vi "Write Device Details.vi"(8 "error in":errorcluster, 10 "Device Details":T1={"Device Port Number"=2001, "Device IP"="192.168.1.1.100", "Timeout"=5000, "Port Number"=1234, "Connection ID"=refnum}, 11 "UDP in":refnum<class "UDP.lvclass">) -> (0 "error out":errorcluster, 3 "UDP out":refnum<class "UDP.lvclass">)   [LabVIEW 2020, in "Plugin Instrument Driver.lvlib" / "UDP.lvclass"]
doc: "Write Device Details"
uses:
  UDP.lvclass
  Typedefs/Device Details.ctl
  UDP.lvclass/UDP.ctl
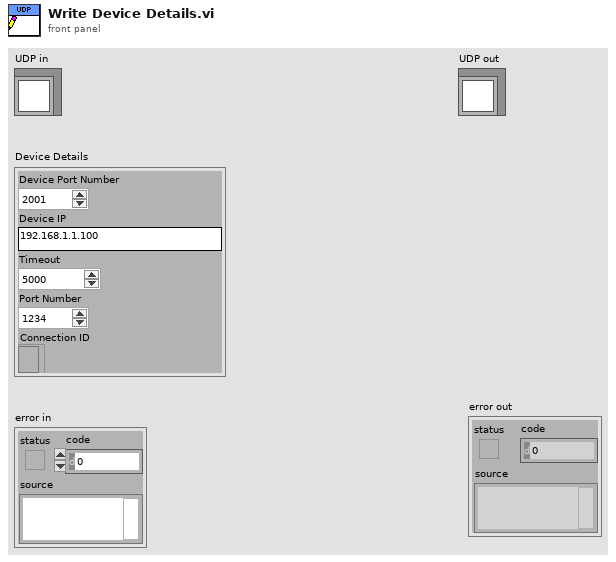
[diagram p1: front panel]
types:
  T1 = typedef "Plugin Instrument Driver.lvlib/UDP.lvclass/Device Details.ctl" = cluster{"Device Port Number":u16, "Device IP":string, "Timeout":i32, "Port Number":u16, "Connection ID":refnum<k16>}
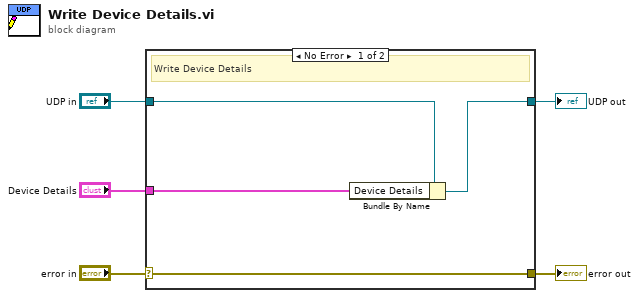
[diagram p0: block diagram]
diagram:
  n1 = case shown="No Error" "error in" {
    selector: "error in" -> [w9 w10]
    tunnel: [w9 w10] -> w4
    tunnel: [w7 w11] -> w2
    tunnel: "UDP in" -> [w8 w11]
    tunnel: "Device Details" -> [w6 _]
    frame No Error {
      # "Write Device Details"
      n2 = Bundle By Name(cluster=w8, "Device Details"=w6) -> (w7:refnum<class "UDP.lvclass">)
    }
    frame Error {
      # "Error"
    }
  }
  "error out" <- w4
  "UDP out" <- w2
